vi "Write Is Parallel.vi"(8 "error in (no error)":errorcluster, 10 "Is Parallel":bool, 11 "USAC Params in":refnum<class "USAC Params.lvclass">) -> (0 "error out":errorcluster, 3 "USAC Params out":refnum<class "USAC Params.lvclass">)   [LabVIEW 2020, in "g_ar_toolkit.ar.lvlib" / "USAC Params.lvclass"]
uses:
  USAC Params.lvclass
  USAC Params.lvclass/USAC Params.ctl
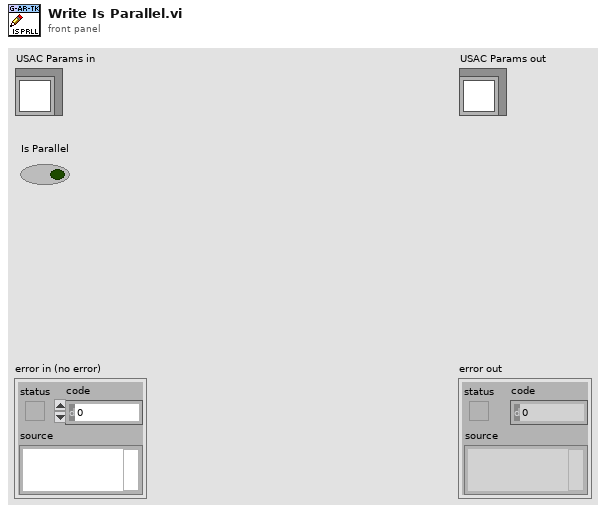
[diagram p1: front panel]
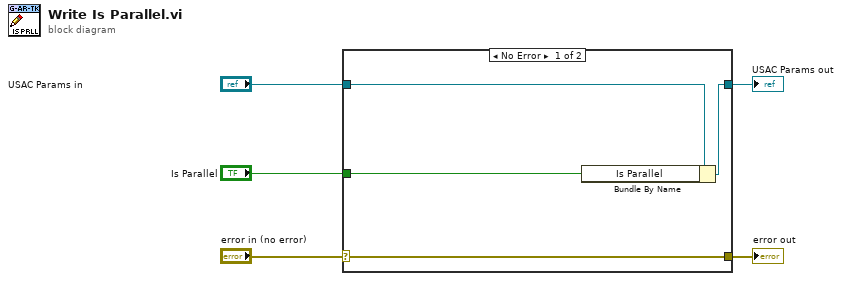
[diagram p0: block diagram]
diagram:
  n1 = case shown="No Error" "error in (no error)" {
    selector: "error in (no error)" -> [w9 w10]
    tunnel: [w9 w10] -> w4
    tunnel: [w7 w11] -> w2
    tunnel: "USAC Params in" -> [w8 w11]
    tunnel: "Is Parallel" -> [w6 _]
    frame No Error {
      n2 = Bundle By Name(cluster=w8, "Is Parallel"=w6) -> (w7:refnum<class "USAC Params.lvclass">)
    }
    frame Error {
    }
  }
  "error out" <- w4
  "USAC Params out" <- w2
